vi "Self Configure.vi"(8 "error in":errorcluster, 11 "SwitchMatrix in":refnum<class "SwitchMatrix.lvclass">) -> (0 "error out":errorcluster, 3 "SwitchMatrix out":refnum<class "SwitchMatrix.lvclass">)   [LabVIEW 2019, in "SwitchMatrix.lvlib" / "SwitchMatrix.lvclass"]
uses:
  Library/SwitchMatrix.lvclass
  Custom Controls/Configuration Keys.ctl
  Library/SwitchMatrix.lvclass/SwitchMatrix.ctl
  builds/Instruments/Instruments.lvlibp/Library/Instruments.lvclass
  builds/Tools/Config.lvlibp/Config.lvclass
  C:/Users/Public/Documents/Development/builds/Tools/Config.lvlibp/Config.lvclass
panel:
  in  "Configuration Keys":T1
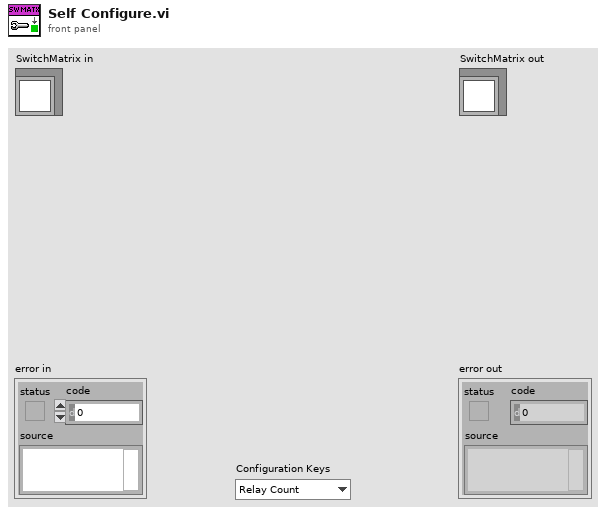
[diagram p1: front panel]
types:
  T1 = typedef "SwitchMatrix.lvlib/SwitchMatrix.lvclass/Configuration Keys.ctl" = enum16{"Relay Count", "Topology"}
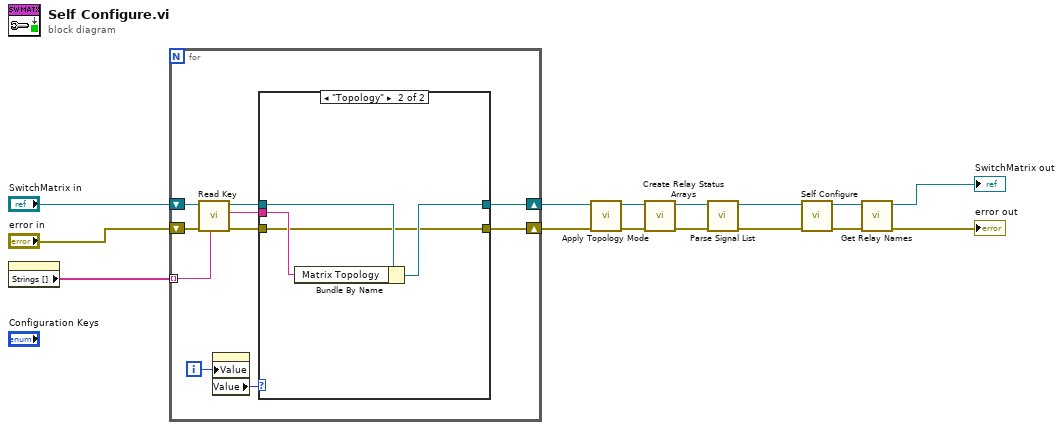
[diagram p0: block diagram]
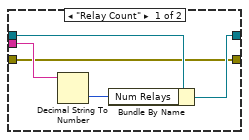
[diagram p2: hidden frame]
diagram:
  n1 = property on="Configuration Keys" class="Enum (strict)"() -> ("Strings []"=w15:string[])  [unwired: 2 in, 2 out]
  n2 = for {
    tunnel: w15 -> [w22] mode=indexing
    shift-right: [w19] -> w8
    shift-left: "SwitchMatrix in" -> [w23]
    shift-right: [w16] -> w7
    shift-left: "error in" -> [w18]
    i -> [w25]
    n3 = call "Read Key.vi"("Key Name"=w22, "error in"=w18, "Config in"=w23) -> ("error out"=w17:errorcluster, "Key Value"=w21:string, "Config out"=w20:refnum<class "SwitchMatrix.lvclass">)  [unwired: 6 in]
    n4 = property on="Configuration Keys" class="Enum (strict)"("Value"=w25) -> ("Value"=w24:T1)  [unwired: 2 in, 2 out]
    n5 = case shown="\"Topology\"" w24 {
      tunnel: w21 -> [w30 w33]
      tunnel: w20 -> [w29 w34]
      tunnel: [w28 w32] -> w19
      tunnel: w17 -> [w26 w31]
      tunnel: [w26 w31] -> w16
      frame "Relay Count" {
        n6 = Decimal String To Number(string=w30) -> (number=w27:i32)  [unwired: 2 in, 1 out]
        n7 = Bundle By Name(cluster=w29, "Num Relays"=w27) -> (w28:refnum<class "SwitchMatrix.lvclass">)
      }
      frame "Topology" {
        n8 = Bundle By Name(cluster=w34, "Matrix Topology"=w33) -> (w32:refnum<class "SwitchMatrix.lvclass">)
      }
    }
  }
  n9 = call "Apply Topology Mode.vi"("error in"=w7, "SwitchMatrix in"=w8) -> ("error out"=w5:errorcluster, "SwitchMatrix out"=w6:refnum<class "SwitchMatrix.lvclass">)  [unwired: 8 in]
  n10 = call "Create Relay Status Arrays.vi"("error in"=w5, "SwitchMatrix in"=w6) -> ("error out"=w3:errorcluster, "SwitchMatrix out"=w4:refnum<class "SwitchMatrix.lvclass">)  [unwired: 8 in]
  n11 = call "Parse Signal List.vi"("error in (no error)"=w3, "SwitchMatrix in"=w4) -> ("error out"=w1:errorcluster, "SwitchMatrix out"=w2:refnum<class "SwitchMatrix.lvclass">)  [unwired: 8 in]
  n12 = call-parent "Self Configure.vi"("error in"=w1, "Instruments in"=w2) -> ("error out"=w12:errorcluster, "Instruments out"=w11:refnum<class "SwitchMatrix.lvclass">)  [unwired: 8 in]
  n13 = call-dynamic "Get Relay Names.vi"("error in (no error)"=w12, "SwitchMatrix in"=w11) -> ("error out"=→"error out":errorcluster, "SwitchMatrix out"=→"SwitchMatrix out":refnum<class "SwitchMatrix.lvclass">)  [unwired: 8 in]
